vi "show workplace data.vi"(9 "輸入":cluster{"條碼A":string, "條碼B":string}[](array[cluster]), 10 "current size":i32, 11 "dimension size":i32) -> (3 "顯示輸出":cluster{"條碼A":string, "條碼B":string}[](array[cluster]))   [LabVIEW 2019]
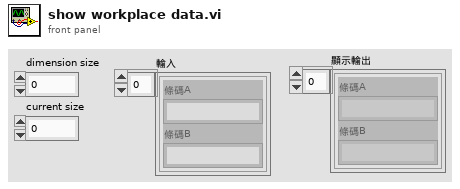
[diagram p1: front panel]
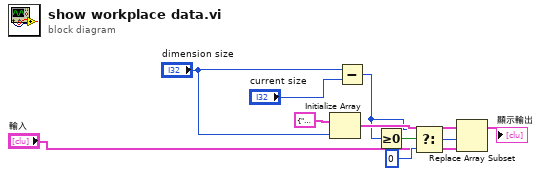
[diagram p0: block diagram]
diagram:
  n1 = Initialize Array(cluster{"條碼A":string, "條碼B":string} {"條碼A"="NULL", "條碼B"="NULL"} ("New data"), "dimension size") -> (w6:cluster{"條碼A":string, "條碼B":string}[])
  n2 = Subtract(x="dimension size", y="current size") -> (x-y=w3:i32)
  n3 = Greater Or Equal To 0?(x=w3) -> (x >= 0?=w8:bool)
  n4 = Select(t=w3, s=w8, f=i16 0) -> (s? t:f=w10:i32)
  n5 = Replace Array Subset(array=w6, new element="輸入", index=w10) -> (→"顯示輸出":cluster{"條碼A":string, "條碼B":string}[])
